vi "Report Status to Caller.vi"(8 "error in":errorcluster, 10 "Status":string, 11 "Customer in":refnum<class "Customer.lvclass">) -> (0 "error out":errorcluster, 3 "Customer out":refnum<class "Customer.lvclass">)   [LabVIEW 2023, in "Customer.lvlib" / "Customer.lvclass"]
doc: "Sends a status message to the higher-level UI for display purposes."
uses:
  Customer.lvclass
  c:/dev/_r/4/eng/lv-core/lvpostprocessingd/lv_mc_x86_64/dist_i386/vi.lib/ActorFramework/Actor/Actor.lvclass
  Coffee Shop/Entity Types.ctl
  <vilib>/ActorFramework/Actor/Actor.lvclass/Actor.ctl
  <vilib>/ActorFramework/Message Enqueuer/Message Enqueuer.lvclass/Message Enqueuer.ctl
  Customer.lvclass/Customer.ctl
  Coffee Shop Messages/Update Entity Details Msg/Update Entity Details Msg.lvclass/Update Entity Details Msg.ctl
  <vilib>/ActorFramework/Message Enqueuer/Init from Existing Queue.vi
  <vilib>/ActorFramework/Message Enqueuer/Enqueue.vi
  Coffee Shop Messages/Update Entity Details Msg/Update Entity Details Msg.lvclass
  c:/dev/_r/4/eng/lv-core/lvpostprocessingd/lv_mc_x86_64/dist_i386/vi.lib/ActorFramework/Message/Message.lvclass
  <vilib>/ActorFramework/Message Priority Queue/Priority Enqueue.vi
  <vilib>/ActorFramework/Message Enqueuer/Message Enqueuer.lvclass
  <vilib>/ActorFramework/Actor/Actor.lvclass
  Coffee Shop/Coffee Shop.lvclass
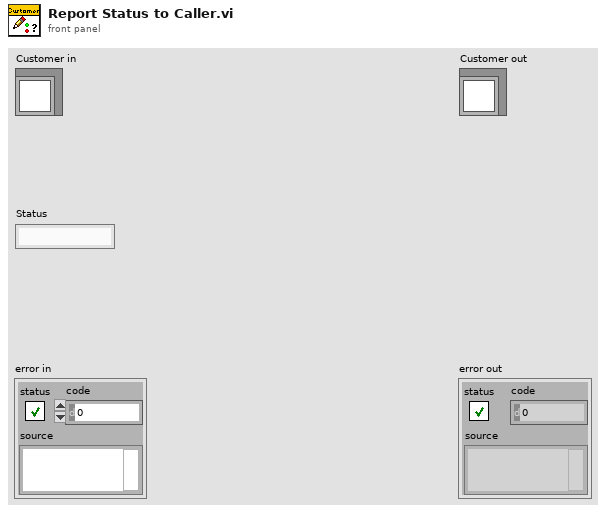
[diagram p1: front panel]
types:
  T1 = typedef "Coffee Shop.lvlib/Coffee Shop.lvclass/Entity Types.ctl" = enum16{"Customer", "Cashier", "Barista"}
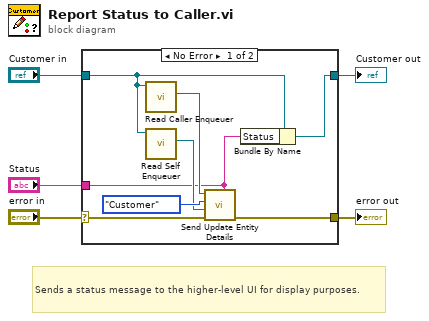
[diagram p0: block diagram]
diagram:
  # "Sends a status message to the higher-level UI for display purposes."
  n1 = case shown="No Error" "error in" {
    selector: "error in" -> [w10 w15]
    tunnel: [w11 w15] -> w4
    tunnel: [w6 w14] -> w2
    tunnel: "Customer in" -> [w8 w14]
    tunnel: "Status" -> [w7 _]
    frame No Error {
      n2 = call <vilib>:"Read Caller Enqueuer.vi"("Actor"=w8) -> ("Caller Enqueuer"=w13:refnum<class "Message Enqueuer.lvclass">)  [unwired: 10 in]
      n3 = call <vilib>:"Read Self Enqueuer.vi"("Actor"=w8) -> ("Self Enqueuer"=w9:refnum<class "Message Enqueuer.lvclass">)  [unwired: 10 in]
      n4 = call "Send Update Entity Details.vi"("status"=w7, "error in (no error)"=w10, "enqueuer"=w9, "Entity Type"=Entity_Types."Customer", "Message Enqueuer"=w13) -> ("error out"=w11:errorcluster)  [unwired: 5 in, 1 out]
      n5 = Bundle By Name(cluster=w8, "Status"=w7) -> (w6:refnum<class "Customer.lvclass">)
    }
    frame Error {
    }
  }
  "error out" <- w4
  "Customer out" <- w2
